vi "finishPreparePassPlay.vi"(8 "error in (no error)":errorcluster, 10 "Game":refnum<class "Game.lvclass">, 11 "PreparePassPlay in":refnum<class "PreparePassPlay.lvclass">) -> (0 "error out":errorcluster, 2 "FinishPreparePass?":bool, 3 "PreparePassPlay out":refnum<class "PreparePassPlay.lvclass">)   [LabVIEW 2023, in "PreparePassPlay.lvclass"]
uses:
  PreparePassPlay.lvclass
  Game_class/Game.lvclass
  Referee_class/command_interpreted.ctl
  Game_class/Game.lvclass/Game.ctl
  Team_class/Team.lvclass/Team.ctl
  Referee_class/Referee.lvclass/Referee.ctl
  Events_class/Events.lvclass/Events.ctl
  Game_class/Read EventsRef.vi
  Events_class/Read ball_out.vi
  Game_class/Read Referee.vi
  Referee_class/Read command_interpreted.vi
  Game_class/Read OffensiveTeam.vi
  Team_class/Read OffensivePlay Finished.vi
  Ally_class/Ally.lvclass
  C:/Users/roboi/Downloads/VSS_AI-Larc2023/Team_class/Team.lvclass
  Referee_class/Referee.lvclass
  Events_class/Events.lvclass
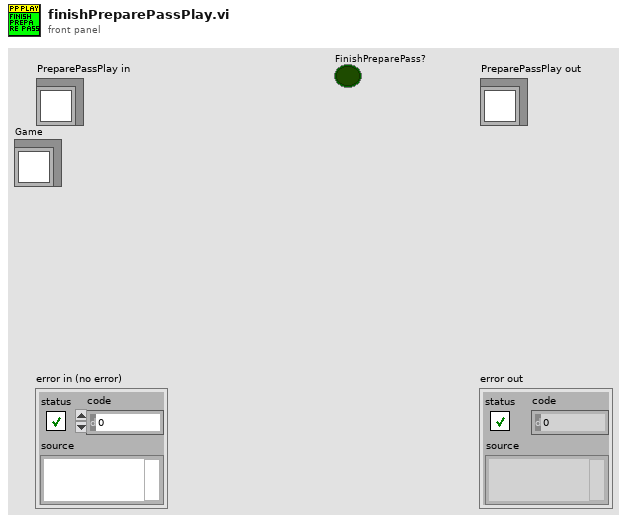
[diagram p1: front panel]
types:
  T1 = typedef "command_interpreted.ctl" = enum16{"Goal Ally", "Goal Enemy", "Ball Placement Enemy", "Ball Placement Ally", "Normal Half Time", "Extra Time  Break", "Extra Half Time", "None", "Post Game", "PKA Normal Start", "Prepare Kickoff Ally", "PKE Normal Start", "Prepare Kickoff Enemy", "Force Start", "Halt", "Timeout", "Prepare Penalty Ally", "Prepare Penalty Enemy", "PPA NormalStart", "PPE Normal Start", "Indirect Free Ally", "Direct Free Enemy", "Direct Free Ally", "Indirect Free Enemy", "Stop"}
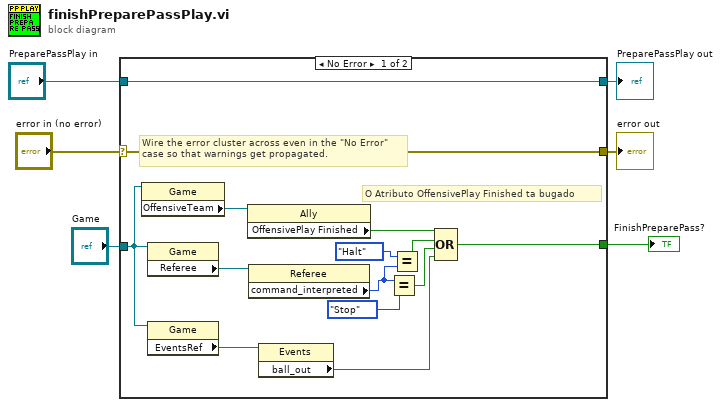
[diagram p0: block diagram]
diagram:
  n1 = case shown="No Error" "error in (no error)" {
    selector: "error in (no error)" -> [w19 w22]
    tunnel: [w19 w22] -> w5
    tunnel: [w20 w21] -> w3
    tunnel: "PreparePassPlay in" -> [w20 w21]
    tunnel: "Game" -> [w16 _]
    tunnel: [w13 _] -> w1
    frame No Error {
      # "O Atributo OffensivePlay Finished ta bugado"
      # "Wire the error cluster across even in the \"No Error\"\ncase so that warnings get propagated."
      n2 = property class="Game"(reference=w16) -> ("OffensiveTeam"=w18:refnum<class "Ally.lvclass">)  [unwired: 1 in, 2 out]
      n3 = property class="Game"(reference=w16) -> ("Referee"=w17:refnum<class "Referee.lvclass">)  [unwired: 1 in, 2 out]
      n4 = property class="Game"(reference=w16) -> ("EventsRef"=w15:refnum<class "Events.lvclass">)  [unwired: 1 in, 2 out]
      n5 = property class="Ally"(reference=w18) -> ("OffensivePlay Finished"=w7:bool)  [unwired: 1 in, 2 out]
      n6 = property class="Referee"(reference=w17) -> ("command_interpreted"=w11:T1)  [unwired: 1 in, 2 out]
      n7 = property class="Events"(reference=w15) -> ("ball_out"=w8:bool)  [unwired: 1 in, 2 out]
      n8 = Equal?(x=w11, y=command_interpreted."Stop") -> (x = y?=w14:bool)
      n9 = Equal?(x=command_interpreted."Halt" ("y"), y=w11) -> (x = y?=w9:bool)
      n10 = Compound Arithmetic op=OR(w7, w9, w14, w8) -> (w13:bool)
    }
    frame Error {
    }
  }
  "error out" <- w5
  "PreparePassPlay out" <- w3
  "FinishPreparePass?" <- w1
